vi "SUB-BLE Rx data Clear.vi"   [LabVIEW 2015]
doc: "Use this template to create an application that executes repeatedly until you click the Stop button. This template polls the state of the Stop button and does not use events. Use the Top-Level Application template (not available in the Base package) to create a single-loop application with event handling."
uses:
  Global 1.vi
panel:
  # "BLE 수신 데이터 버퍼 리셋"
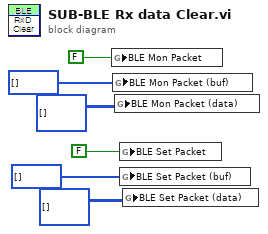
[diagram p0: block diagram]
diagram:
  n1 = global write "Global 1.vi" "BLE Mon Packet"(FALSE ("BLE Packet")) -> ()
  n2 = global write "Global 1.vi" "BLE Mon Packet (buf)"(u8[] [] ("BLE Packet (buf)")) -> ()
  n3 = global write "Global 1.vi" "BLE Mon Packet (data)"(u8[][] [] ("BLE Packet (data)")) -> ()
  n4 = global write "Global 1.vi" "BLE Set Packet"(FALSE ("BLE Packet")) -> ()
  n5 = global write "Global 1.vi" "BLE Set Packet (buf)"(u8[] [] ("BLE Packet (buf)")) -> ()
  n6 = global write "Global 1.vi" "BLE Set Packet (data)"(u8[][] [] ("BLE Packet (data)")) -> ()
